vi "Create Evaluations.vi"(8 "error in (no error)":errorcluster, 11 "IEvaluation in":refnum<class "HiSi_SpecAn_IQSLOT.lvclass">) -> (0 "error out":errorcluster, 2 "Evaluations Out":T1[](array[typedef]) {"Low Limit" format="%#_13g"; "SI Scaling" items=["femto"=-15, "pico"=-12, "nano"=-9, "micro"=-6, "milli"=-3, "percent"=-2, ""=0, "kilo"=3, "mega"=6, "giga"=9, "tera"=12]}, 3 "IEvaluation out":refnum<class "HiSi_SpecAn_IQSLOT.lvclass">)   [LabVIEW 2018, in "SeqAuto Evaluations.lvlib" / "HiSi_SpecAn_IQSLOT.lvclass"]
uses:
  HiSi_SpecAn_IQSLOT.lvclass
  C:/Sequence Automation/Plugins/SeqAuto IEvaluation.lvlibp/SeqAuto IEvaluation.lvclass
  Plugins/TestStand API Tools (TSAT).lvlibp/Evaluation Actions/Includes/Controls/TSAT Evaluation.ctl
  Plugins/TestStand API Tools (TSAT).lvlibp/Evaluation Actions/Includes/Controls/TSAT Eval SI Unit Scaling.ctl
  Plugins/TestStand API Tools (TSAT).lvlibp/Evaluation Actions/Includes/Controls/TSAT Evaluation Type.ctl
  HiSi_SpecAn_IQSLOT.lvclass/HiSi_SpecAn_IQSLOT.ctl
  Plugins/SeqAuto IEvaluation.lvlibp/Read Measurement Name.vi
  Plugins/TestStand API Tools (TSAT).lvlibp/Evaluation Actions/TSAT Evaluation Actions.lvlib
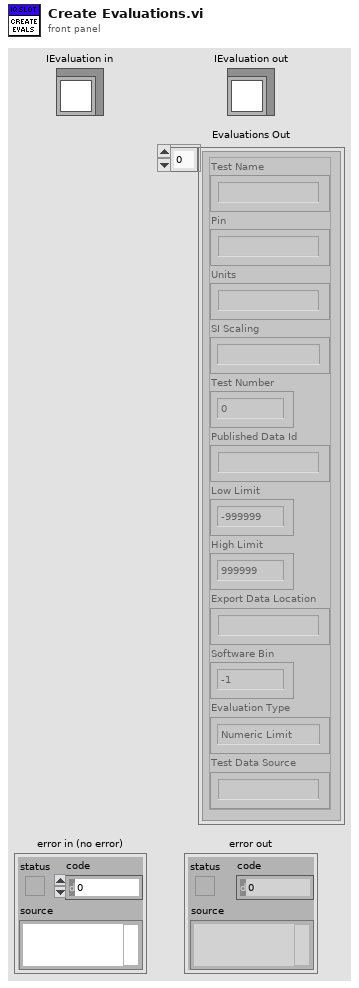
[diagram p1: front panel]
types:
  T1 = typedef "TestStand API Tools (TSAT).lvlibp/TSAT Evaluation Actions.lvlib/TSAT Evaluation.ctl" = cluster{"Test Name":string, "Pin":string, "Units":string, "SI Scaling":T2, "Test Number":i32, "Published Data Id":string, "Low Limit":dbl, "High Limit":dbl, "Export Data Location":string, "Software Bin":i64, "Evaluation Type":T3, "Test Data Source":string}
  T2 = typedef "TestStand API Tools (TSAT).lvlibp/TSAT Evaluation Actions.lvlib/TSAT Eval SI Unit Scaling.ctl" = i16
  T3 = typedef "TestStand API Tools (TSAT).lvlibp/TSAT Evaluation Actions.lvlib/TSAT Evaluation Type.ctl" = enum16{"Numeric Limit", "Pass/Fail", "None"}
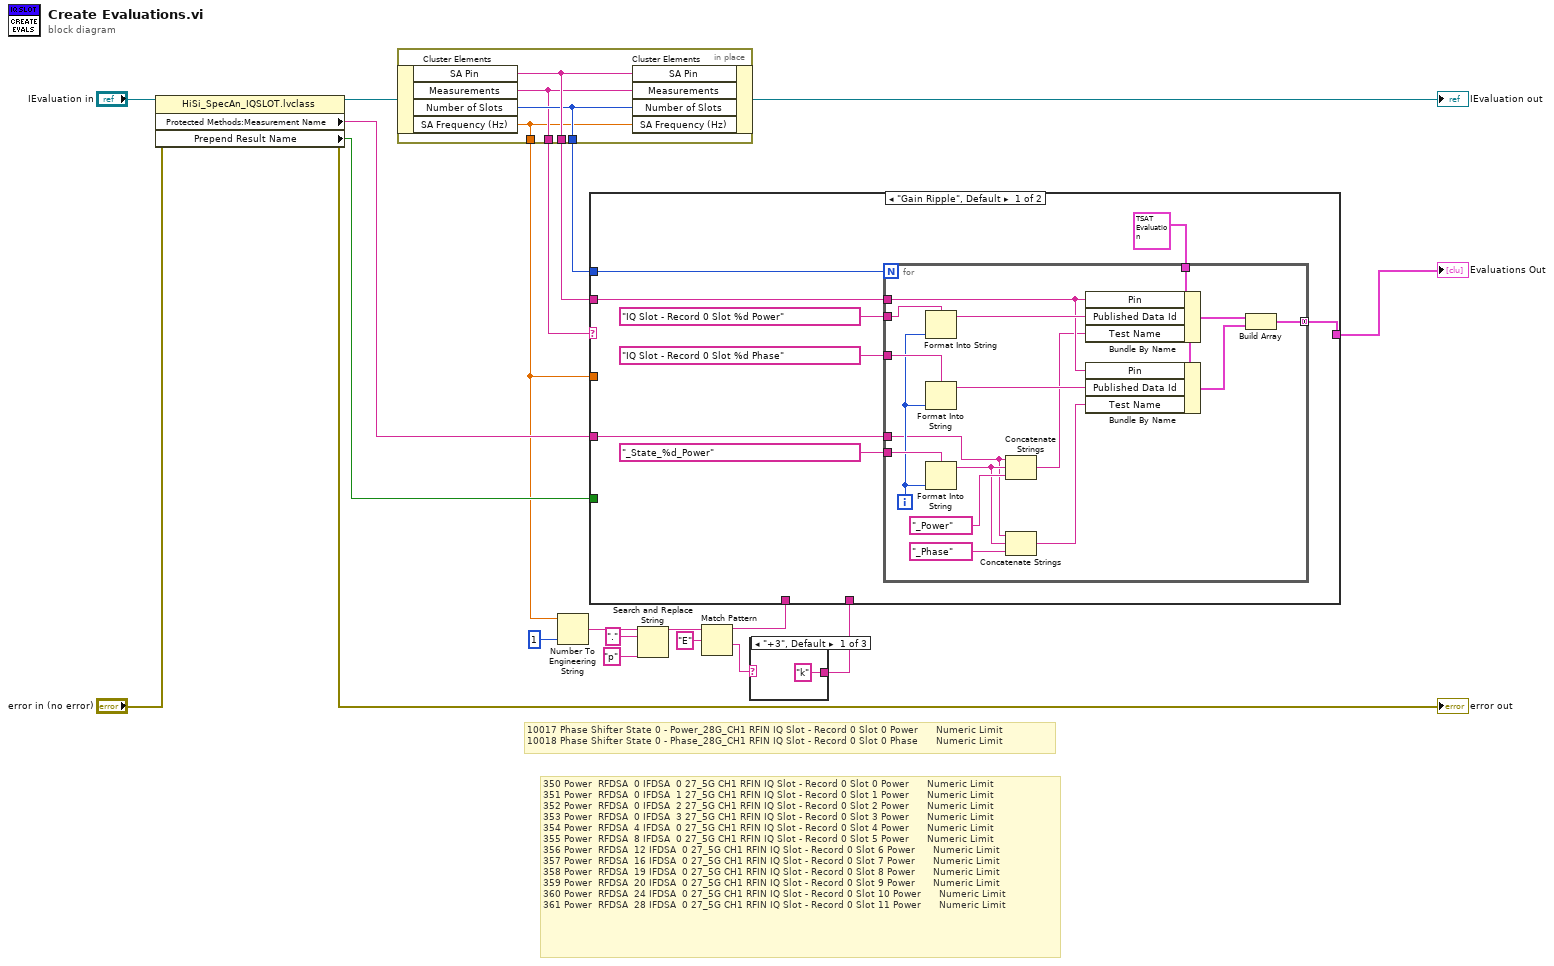
[diagram p0: block diagram]
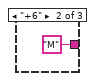
[diagram p2: hidden frame]
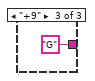
[diagram p3: hidden frame]
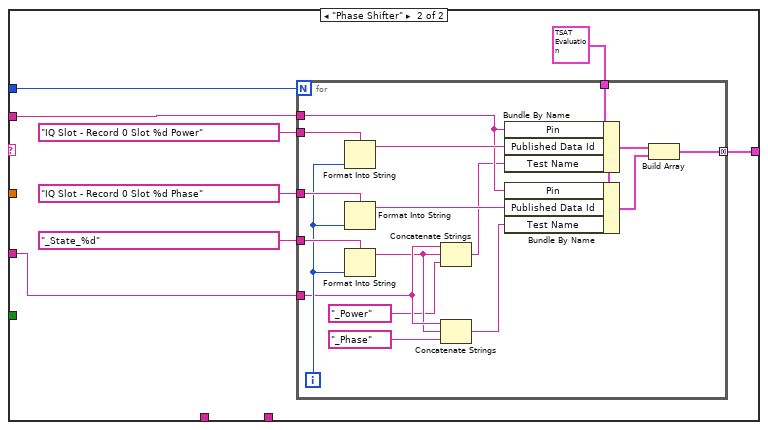
[diagram p4: hidden frame]
diagram:
  # "350\tPower  RFDSA  0 IFDSA  0 27_5G CH1\tRFIN\tIQ Slot - Record 0 Slot 0 Power\t\t\t\t\t\tNumeric Limit\t\t\n351\tPower  RFDSA  0 IFDSA  1 27_5G CH1\tRFIN\tIQ Slot - Record 0 Slot 1 Power\t\t\t\t\t\tNumeric Limit\t\t\n352\tPower  RFDSA  0 IFDSA  2 27_5G CH1\tRFIN\tIQ Slot - Record 0 Slot 2 Power\t\t\t\t\t\tNumeric Limit\t\t\n353\tPower  RFDSA  0 IFDSA  3 27_5G CH1\tRFIN\tIQ Slot - Record 0 Slot 3 Power\t\t\t\t\t\tNumeric Limit\t\t\n354\tPower  RFDSA  4 IFDSA  0 27_5G CH1\tRFIN\tIQ Slot - Record 0 Slot 4 Power\t\t\t\t\t\tNumeric Limit\t\t\n355\tPower  RFDSA  8 IFDSA  0 27_5G CH1\tRFIN\tIQ Slot - Record 0 Slot 5 Power\t\t\t\t\t\tNumeric Limit\t\t\n356\tPower  RFDSA  12 IFDSA  0 27_5G CH1\tRFIN\tIQ Slot - Record 0 Slot 6 Power\t\t\t\t\t\tNumeric Limit\t\t\n357\tPower  RFDSA  16 IFDSA  0 27_5G CH1\tRFIN\tIQ Slot - Record 0 Slot 7 Power\t\t\t\t\t\tNumeric Limit\t\t\n358\tPower  RFDSA  19 IFDSA  0 27_5G CH1\tRFIN\tIQ Slot - Record 0 Slot 8 Power\t\t\t\t\t\tNumeric Limit\t\t\n359\tPower  RFDSA  20 IFDSA  0 27_5G CH1\tRFIN\tIQ Slot - Record 0 Slot 9 Power\t\t\t\t\t\tNumeric Limit\t\t\n360\tPower  RFDSA  24 IFDSA  0 27_5G CH1\tRFIN\tIQ Slot - Record 0 Slot 10 Power\t\t\t\t\t\tNumeric Limit\t\t\n361\tPower  RFDSA  28 IFDSA  0 27_5G CH1\tRFIN\tIQ Slot - Record 0 Slot 11 Power\t\t\t\t\t\tNumeric Limit"
  # "10017\tPhase Shifter State 0 - Power_28G_CH1\tRFIN\tIQ Slot - Record 0 Slot 0 Power\t\t\t\t\t\tNumeric Limit\t\t\n10018\tPhase Shifter State 0 - Phase_28G_CH1\tRFIN\tIQ Slot - Record 0 Slot 0 Phase\t\t\t\t\t\tNumeric Limit"
  n1 = property class="HiSi_SpecAn_IQSLOT.lvclass"(reference="IEvaluation in", error in="error in (no error)") -> (reference out=w19:refnum<class "HiSi_SpecAn_IQSLOT.lvclass">, error out=→"error out":errorcluster, "Protected Methods:Measurement Name"=w14:string, "Prepend Result Name"=w13:bool)
  n2 = in-place {
    in-place-border: [w25] -> w15
    in-place-border: [w24] -> w12
    in-place-border: [w23] -> w11
    in-place-border: [w22] -> w4
    n3 = in-place-cluster #1(w19) -> ("SA Pin"=w25:string, "Measurements"=w23:string, "Number of Slots"=w24:i32, "SA Frequency (Hz)"=w22:dbl)
    n4 = in-place-cluster #1("SA Pin"=w25, "Measurements"=w23, "Number of Slots"=w24, "SA Frequency (Hz)"=w22) -> (→"IEvaluation out":refnum<class "HiSi_SpecAn_IQSLOT.lvclass">)
  }
  n5 = Number To Engineering String(2:i16 1 ("precision (6)"), 4:w4) -> (0:w9:string)  [unwired: 2 in]
  n6 = Search and Replace String(input string=w9, search string=".", replace string="p" ("replace string (\"\")")) -> (result string=w6:string)  [unwired: 5 in, 3 out]
  n7 = Match Pattern(string=w6, regular expression="E") -> (before substring=w3:string, after substring=w2:string)  [unwired: 1 in, 2 out]
  n8 = case shown="\"+3\", Default" w2 {
    tunnel: ["k" ("regular expression") "M" ("regular expression") "G" ("regular expression")] -> w1
    frame "+3", Default {
    }
    frame "+6" {
    }
    frame "+9" {
    }
  }
  n9 = case shown="\"Gain Ripple\", Default" w11 {
    tunnel: [w36 w61] -> w18
    tunnel: w15 -> [w34 w59]
    tunnel: w14 -> [w29 w54]
    tunnel: w13 -> [_ _]
    tunnel: w12 -> [w33 w58]
    tunnel: w4 -> [_ _]
    tunnel: w3 -> [_ _]
    tunnel: w1 -> [_ _]
    frame "Gain Ripple", Default {
      n10 = for {
        N: w33 -> [_]
        tunnel: "IQ Slot - Record 0 Slot %d Power" -> [w51]
        tunnel: T1 {"Test Name"="", "Pin"="", "Units"="", "SI Scaling"=0, "Test Number"=0, "Published Data Id"="", "Low Limit"=-999999.0, "High Limit"=999999.0, "Export Data Location"="", "Software Bin"=-1, "Evaluation Type"=enum."Numeric Limit", "Test Data Source"=""} ("Evaluation") -> [w47]
        tunnel: [w46] -> w36 mode=concatenating
        tunnel: w34 -> [w49]
        tunnel: "IQ Slot - Record 0 Slot %d Phase" -> [w50]
        tunnel: "_State_%d_Power" -> [w44]
        tunnel: w29 -> [w37]
        i -> [w42]
        n11 = Format Into String(format string=w51, w42) -> (resulting string=w53:string)  [unwired: 2 in, 1 out]
        n12 = Format Into String(format string=w50, w42) -> (resulting string=w48:string)  [unwired: 2 in, 1 out]
        n13 = Format Into String(format string=w44, w42) -> (resulting string=w39:string)  [unwired: 2 in, 1 out]
        n14 = Concatenate Strings(w37, w39, "_Power") -> (w43:string)
        n15 = Concatenate Strings(w37, w39, "_Phase") -> (w38:string)
        n16 = Bundle By Name(cluster=w47, "Pin"=w49, "Published Data Id"=w53, "Test Name"=w43) -> (w52:T1)
        n17 = Bundle By Name(cluster=w47, "Pin"=w49, "Published Data Id"=w48, "Test Name"=w38) -> (w45:T1)
        n18 = Build Array(w52, w45) -> (w46:T1[])
      }
    }
    frame "Phase Shifter" {
      n19 = for {
        N: w58 -> [_]
        tunnel: "IQ Slot - Record 0 Slot %d Power" -> [w76]
        tunnel: T1 {"Test Name"="", "Pin"="", "Units"="", "SI Scaling"=0, "Test Number"=0, "Published Data Id"="", "Low Limit"=-999999.0, "High Limit"=999999.0, "Export Data Location"="", "Software Bin"=-1, "Evaluation Type"=enum."Numeric Limit", "Test Data Source"=""} ("Evaluation") -> [w72]
        tunnel: [w71] -> w61 mode=concatenating
        tunnel: w59 -> [w74]
        tunnel: "IQ Slot - Record 0 Slot %d Phase" -> [w75]
        tunnel: "_State_%d" -> [w69]
        tunnel: w54 -> [w67]
        i -> [w68]
        n20 = Format Into String(format string=w76, w68) -> (resulting string=w78:string)  [unwired: 2 in, 1 out]
        n21 = Format Into String(format string=w75, w68) -> (resulting string=w73:string)  [unwired: 2 in, 1 out]
        n22 = Format Into String(format string=w69, w68) -> (resulting string=w64:string)  [unwired: 2 in, 1 out]
        n23 = Concatenate Strings(w67, w64, "_Power") -> (w65:string)
        n24 = Concatenate Strings(w67, w64, "_Phase") -> (w66:string)
        n25 = Bundle By Name(cluster=w72, "Pin"=w74, "Published Data Id"=w78, "Test Name"=w65) -> (w77:T1)
        n26 = Bundle By Name(cluster=w72, "Pin"=w74, "Published Data Id"=w73, "Test Name"=w66) -> (w70:T1)
        n27 = Build Array(w77, w70) -> (w71:T1[])
      }
    }
  }
  "Evaluations Out" <- w18
